vi "Get All Fault Configurations.vi"(8 "error in (no error)":errorcluster, 11 "target address (localhost)":string="localhost") -> (0 "error out":errorcluster, 3 "configured faults":T1[](array[typedef]) {"level after threshold" items=["Ignore"=-1, "Minor"=0, "Major"=1]; "level or level before threshold" items=["Ignore"=-1, "Minor"=0, "Major"=1]})   [LabVIEW 2020, in "Config Faults.lvlib"]
doc: "Returns a list of custom fault configurations."
uses:
  <vilib>/NIScanEngine/ConfigurableFaults/Config Faults.lvlib
  <vilib>/NIScanEngine/ConfigurableFaults/Fault Desc Control.ctl
  <resource>/objmgr/ni.var.rc
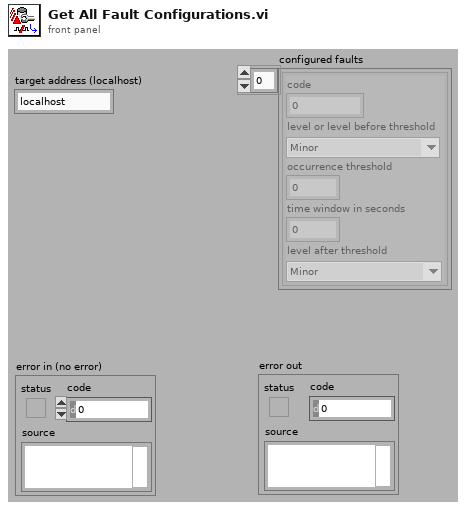
[diagram p1: front panel]
types:
  T1 = typedef "Config Faults.lvlib/Fault Desc Control.ctl" = cluster{"code":i32, "level or level before threshold":i32, "occurrence threshold":u32, "time window in seconds":u32, "level after threshold":i32}
  T2 = typedef "Fault Desc Control.ctl" = cluster{"code":i32, "level or level before threshold":i32, "occurrence threshold":u32, "time window in seconds":u32, "level after threshold":i32}
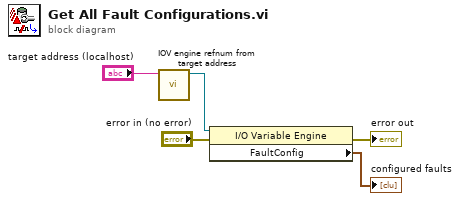
[diagram p0: block diagram]
diagram:
  n1 = call <vilib>:"IOV engine refnum from target address.vi"("target address"="target address (localhost)") -> ("reference out"=w5:refnum<k21>)  [unwired: 10 in]
  n2 = property class="I/O Variable Engine"(reference=w5, error in="error in (no error)") -> (error out=→"error out":errorcluster, "FaultConfig"=→"configured faults":T2[])  [unwired: 1 out]
